vi "Open_Instr.vi"(8 "error in (no error)":errorcluster caption="entrée d'erreur (pas d'erreur)", 11 "Class Multimeter Multimeter en entrée":refnum<class "Class Instrument LED_Analyser.lvclass">) -> (0 "error out":errorcluster caption="sortie d'erreur", 3 "Class Multimeter Multimeter en sortie":refnum<class "Class Instrument LED_Analyser.lvclass">)   [LabVIEW 2020, in "Library Instrument & Equipement.lvlib" / "Library Instruments.lvlib" / "Class Instrument LED_Analyser.lvclass"]
uses:
  Class Instrument LED_Analyser.lvclass
  Class Instrument LED_Analyser.lvclass/Class Instrument LED_Analyser.ctl
  Instrument (Default)/Class Instrument (Default).lvclass
  LED Analyser/Class Led Analyser (Default)/Class LED Analyser (Default).lvclass
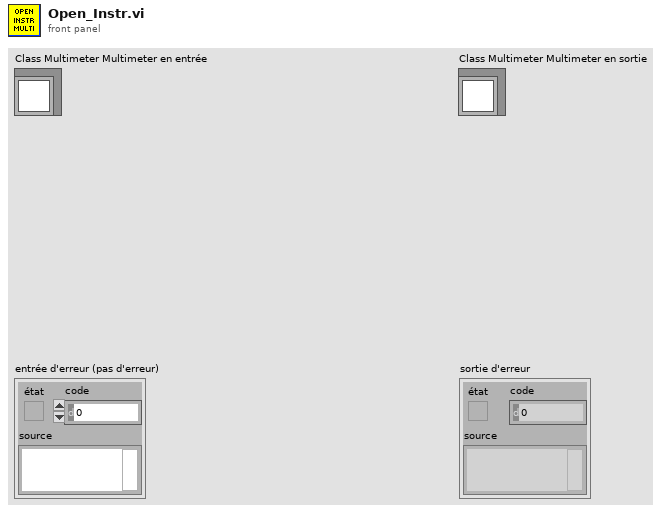
[diagram p1: front panel]
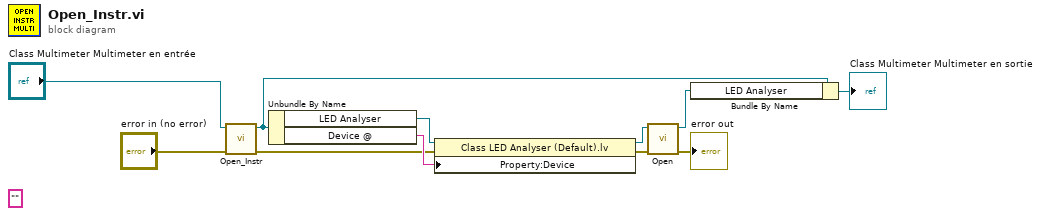
[diagram p0: block diagram]
diagram:
  (unwired) "" ("Device")
  n1 = call-parent "Open_Instr.vi"("error in (no error)"="error in (no error)", "Class Multimeter (Default) en entrée"="Class Multimeter Multimeter en entrée") -> ("error out"=w4:errorcluster, "Class Multimeter (Default) en sortie"=w8:refnum<class "Class Instrument LED_Analyser.lvclass">)  [unwired: 8 in]
  n2 = Unbundle By Name(w8) -> ("LED Analyser"=w3:refnum<class "Class LED Analyser (Default).lvclass">, "Device @"=w5:string)
  n3 = property class="Class LED Analyser (Default).lv"(reference=w3, error in=w4, "Property:Device"=w5) -> (reference out=w1:refnum<class "Class LED Analyser (Default).lvclass">, error out=w2:errorcluster)
  n4 = call-dynamic "Open.vi"("error in (no error)"=w2, "Class LED Analyser in"=w1) -> ("error out"=→"error out":errorcluster, "Class LED Analyser Out"=w7:refnum<class "Class LED Analyser (Default).lvclass">)  [unwired: 8 in]
  n5 = Bundle By Name(cluster=w8, "LED Analyser"=w7) -> (→"Class Multimeter Multimeter en sortie":refnum<class "Class Instrument LED_Analyser.lvclass">)
